vi "Periodic Tasks.vi"(8 "error in":errorcluster) -> ()   [LabVIEW 2016]
doc: "This VI runs in parallel to other tasks. It can contain as many user-defined periodic loops as you need. These can carry out PID or other sorts of timed response."
uses:
  <userlib>/836-libraries/Drive/Drive_Code_V2/Drive_Code_Support/PidClusters/Drive_Code_PID_Bundle.ctl
  <userlib>/836-libraries/Drive/Drive_Code_V2/Drive_Code_Support/Command_Sends/Drive_Code_Command_List.ctl
  <userlib>/836-libraries/Drive/Drive_Code_V2/Drive_Code_Support/SensorTypedefs/Sensor_Cluster.ctl
  <userlib>/836-libraries/Drive/Drive_Code_V2/Drive_Code_Support/SensorTypedefs/Camera_Cluster.ctl
  <vilib>/Rock Robotics/WPI/RobotDrive/WPI_RobotDriveDevRef.ctl
  <vilib>/Rock Robotics/WPI/MotorControl/WPI_MotorControlDeviceRef.ctl
  <vilib>/Rock Robotics/WPI/MotorControl/WPI_MotorControlType.ctl
  <vilib>/Rock Robotics/SystemInterfaces/DIO/FPGA_DIOPWMChannel.ctl
  <vilib>/Rock Robotics/WPI/PWM/WPI_PWMDeadband.ctl
  <userlib>/836-libraries/Drive/Drive_Code_V2/Drive_Code_Support/DriveTrains/Drive_Trains.ctl
  <userlib>/836-libraries/Drive/Drive_Code_V2/Drive_Code_Support/Command_Sends/Drive_Code_Command_Type.ctl
  <userlib>/836-libraries/Drive/Drive_Code_V2/Drive_Code_Support/PidClusters/PidInversions.ctl
  <vilib>/Platform/TimedLoop/XDataNode/timing_clust.ctl
  <vilib>/Platform/TimedLoop/XDataNode/nitl_modes.ctl
  <vilib>/Platform/TimedLoop/XDataNode/wakeup.ctl
  <vilib>/Rock Robotics/WPI/Utilities/WPI_GetSetVariantRefNum.vi
  <userlib>/836-libraries/Drive/Drive_Code_V2/Drive_Code_Support/Command_Sends/Drive_Cmd_Cheesey_Drive.vi
  <userlib>/836-libraries/Drive/Drive_Code_V2/Drive_Code_Support/Command_Sends/Drive_Cmd_Drive_Continuous.vi
  <userlib>/836-libraries/Drive/Drive_Code_V2/Drive_Code_Support/Command_Sends/Drive_Cmd_Turn.vi
  <userlib>/836-libraries/Drive/Drive_Code_V2/Drive_Code_Support/Command_Sends/Drive_Cmd_Drive_Distance.vi
  <userlib>/836-libraries/Drive/Drive_Code_V2/Drive_Code_Support/Command_Sends/Drive_Cmd_Hold_Position.vi
  <userlib>/836-libraries/Drive/Drive_Code_V2/Drive_Code_Support/Command_Sends/Drive_Cmd_Hold_Yaw.vi
  <userlib>/836-libraries/Drive/Drive_Code_V2/Drive_Code_Support/Command_Sends/Drive_Cmd_PID_Update.vi
  <userlib>/836-libraries/Drive/Drive_Code_V2/Drive_Code_Support/Command_Sends/Drive_Cmd_Update_Period.vi
  <userlib>/836-libraries/Drive/Drive_Code_V2/Drive_Code_Support/Command_Sends/Drive_Cmd_Update_PID_Inversion.vi
  <vilib>/platform/TimedLoop/XDataNode/XDataNode.xnode
  <vilib>/Platform/TimedLoop/XDataNode/XDNodeRunTimeDep.lvlib
panel:
  out "SensorFinishedLate":bool
  out "Drive Finished Late":bool
  in  "Tab Control":enum32{"Drive", "Sensors"}(tab)
  out "Distance Error":dbl(knob) scale=0.0..3.0
  out "Turn Error":dbl(knob) scale=0.0..3.0
  in  "Distance Absolute?":bool
  in  "Desired Distance":dbl
  in  "Angle Absolute?":bool
  in  "Desired Angle":dbl
  in  "Max Distance Power":dbl(knob) scale=0.0..1.0
  in  "Max Turn Power":dbl(knob) scale=0.0..1.0
  out "PID Response Turn":cluster{"Yaw":dbl, "Desired Angle":dbl}(graph)
  out "PID Response Distance":cluster{"Distance":dbl, "Desired Distance":dbl}(graph)
  in  "PID Gains":T1={"Yaw, Driving Straight"={"proportional gain (Kc)"=0.025, "integral time (Ti, min)"=0.0, "derivative time (Td, min)"=0.0}, "Yaw, Holding Still"={"proportional gain (Kc)"=0.027, "integral time (Ti, min)"=0.0125, "derivative time (Td, min)"=0.0}, "Distance, Driving Straight"={"proportional gain (Kc)"=1.0, "integral time (Ti, min)"=0.5, "derivative time (Td, min)"=0.0}, "Distance, Holding Still"={"proportional gain (Kc)"=1.0, "integral time (Ti, min)"=0.01, "derivative time (Td, min)"=0.0}}
  in  "Command":T2
  in  "Yaw PID Inverted?":bool
  in  "Distance PID Inverted?":bool
  out "Roll":dbl(graph)
  out "Pitch":dbl(graph)
  out "Yaw":dbl(graph)
  out "Distance":dbl(graph)
  in  "Read Enable":T3={"Cal Status"=TRUE, "Orientation"=TRUE, "Gyro"=FALSE, "Accelerometer"=FALSE, "Quanterion"=FALSE, "Accel Mode"=enum."Linear", "Magnetometer"=FALSE, "Register Mode"=enum."Quaternion"}
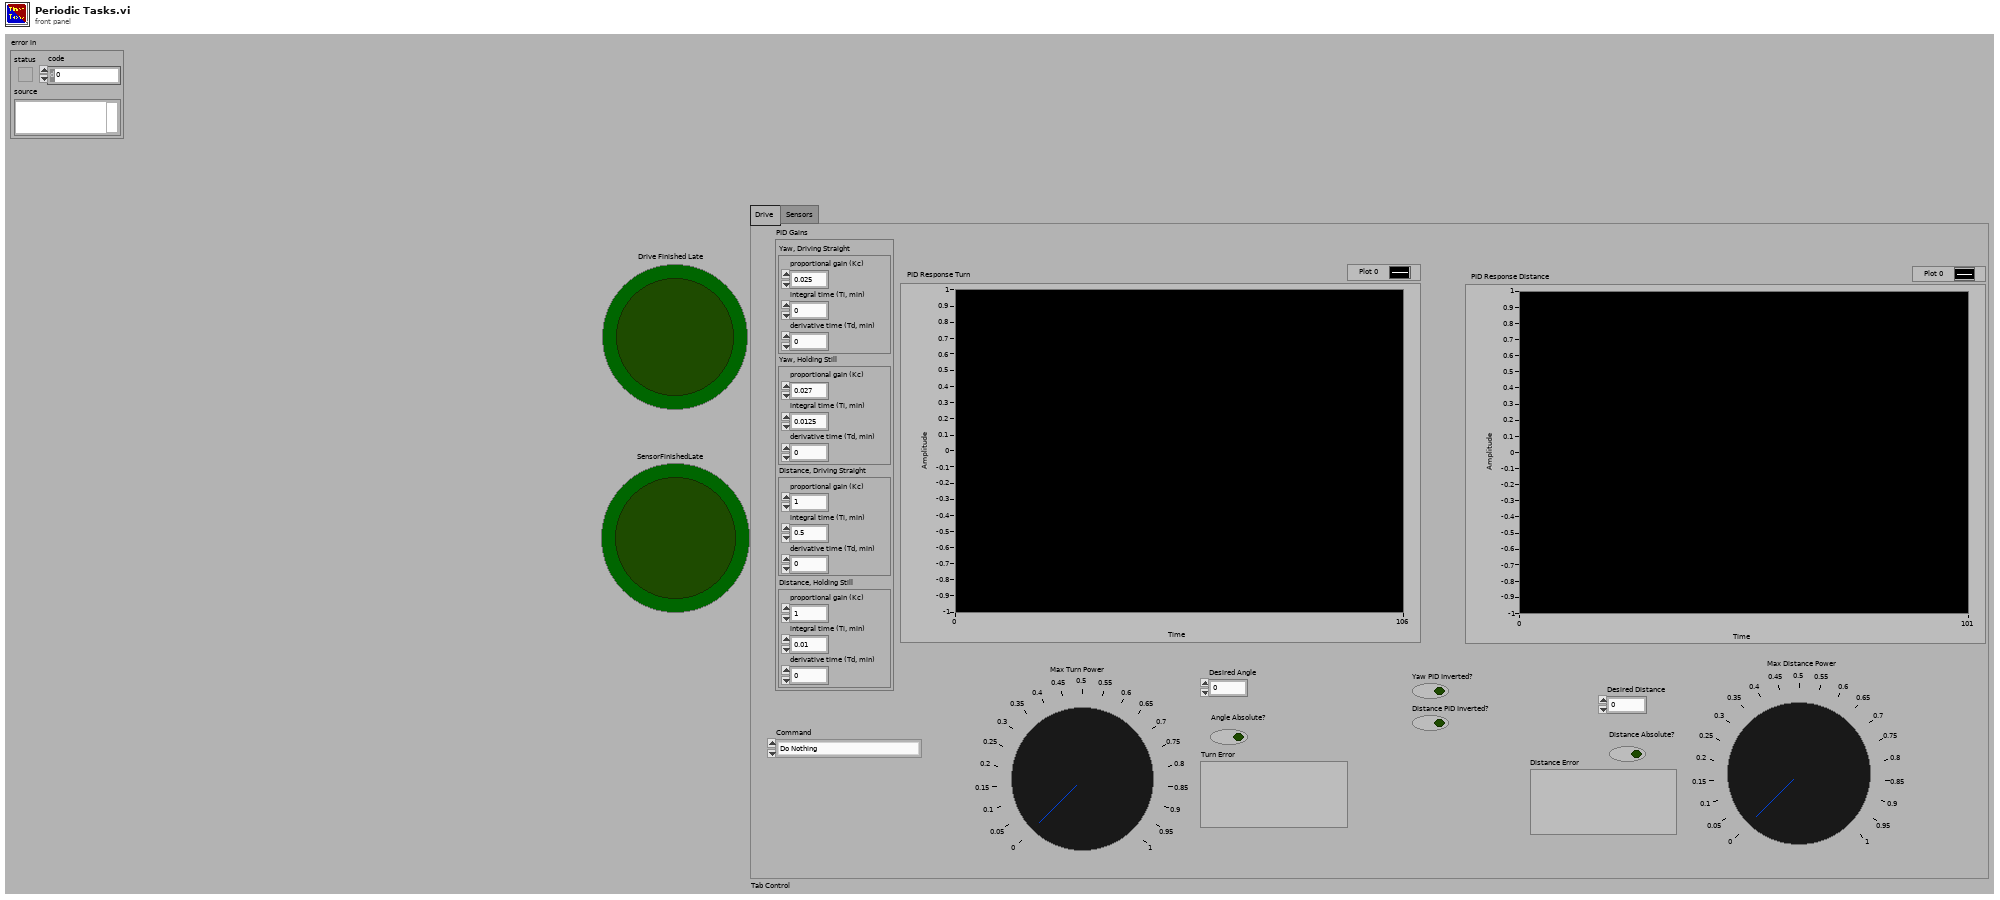
[diagram p1: front panel]
types:
  T1 = typedef "Drive_Code_PID_Bundle.ctl" = cluster{"Yaw, Driving Straight":cluster{"proportional gain (Kc)":dbl, "integral time (Ti, min)":dbl, "derivative time (Td, min)":dbl}, "Yaw, Holding Still":cluster{"proportional gain (Kc)":dbl, "integral time (Ti, min)":dbl, "derivative time (Td, min)":dbl}, "Distance, Driving Straight":cluster{"proportional gain (Kc)":dbl, "integral time (Ti, min)":dbl, "derivative time (Td, min)":dbl}, "Distance, Holding Still":cluster{"proportional gain (Kc)":dbl, "integral time (Ti, min)":dbl, "derivative time (Td, min)":dbl}}
  T2 = typedef "Drive_Code_Command_List.ctl" = enum16{"Do Nothing", "Tank Drive", "Drive Continuous", "Turn", "Drive Distance", "Hold Position", "Hold Yaw", "Follow Camera", "Turn to Camera", "Approach Camera", "PID Update", "Cheesy Drive", "Update Period", "Update PID Inversions"}
  T3 = cluster{"Cal Status":bool, "Orientation":bool, "Gyro":bool, "Accelerometer":bool, "Quanterion":bool, "Accel Mode":enum8{"Raw Data", "Linear", "Gravity"}, "Magnetometer":bool, "Register Mode":enum8{"Euler", "Quaternion"}}
  T4 = typedef "Sensor_Cluster.ctl" = cluster{"Gyro Data":cluster{"Gyro RT FIFO":refnum<k33>, "Gyro Current":dbl, "Gyro Hold":dbl}, "Encoder Data":cluster{"Encoder RT FIFO":refnum<k33>, "Encoder Current":dbl, "Encoder Hold":dbl}, "Camera Data":cluster{"Camera RT FIFO":refnum<k33>, "Camera Current":T5}}
  T5 = typedef "Camera_Cluster.ctl" = cluster{" Angle":dbl, "Valid":bool}
  T6 = typedef "WPI_RobotDriveDevRef.ctl" = cluster{"DevStatus":errorcluster, "Motors[]":T7[], "Square Inputs":bool, "Max Output":dbl}
  T7 = typedef "WPI_MotorControlDeviceRef.ctl" = cluster{"DeviceStatus":errorcluster, "Type":T8, "PWM":cluster{"PWM Channel":T9, "DeadBand":T10}, "CAN":cluster{"Device Number":u8, "SetOutput VI Ref":variant, "GetOutput VI Ref":variant, "Enable VI Ref":variant, "Disable VI Ref":variant, "Data":variant}, "Invert":bool}
  T8 = typedef "WPI_MotorControlType.ctl" = enum16{"PWM", "CAN"}
  T9 = typedef "FPGA_DIOPWMChannel.ctl" = enum8{"PWM 0", "PWM 1", "PWM 2", "PWM 3", "PWM 4", "PWM 5", "PWM 6", "PWM 7", "PWM 8", "PWM 9", "PWM MXP 0", "PWM MXP 1", "PWM MXP 2", "PWM MXP 3", "PWM MXP 4", "PWM MXP 5", "PWM MXP 6", "PWM MXP 7", "PWM MXP 8", "PWM MXP 9", "Invalid"}
  T10 = typedef "WPI_PWMDeadband.ctl" = cluster{"Name":string, "maxPositivePwm":i32, "minPositivePwm":i32, "centerPwm":i32, "maxNegativePwm":i32, "minNegativePwm":i32, "angularRange":u16}
  T11 = typedef "Drive_Trains.ctl" = enum16{"Tank Drive 2 Motor", "Tank Drive 4 Motor", "Mecanum Drive", "Kiwi Drive"}
  T12 = typedef "PidInversions.ctl" = cluster{"Distance PID Inverted?":bool, "Yaw PID Inverted?":bool}
  T13 = cluster{"Sensor Data":T4, "RobotDriveDevRef":T6, "Drive Train":T11, "Valid Commands":bool[], "Drive Comand Notifier":refnum<notifier>, "Command Finished?":refnum<k4>, "Command Canceled":refnum<k4>, "PID Inversions":T12}
  T14 = typedef "WPI_JoystickDevRef.ctl" = cluster{"Device":T15}
  T15 = typedef "WPI_JoystickDeviceEnum.ctl" = enum16{"USB 0", "USB 1", "USB 2", "USB 3", "USB 4", "USB 5"}
  T16 = typedef "XDNodeRunTimeDep.lvlib/timing_clust.ctl" = cluster{"Expected End [f-1]":u64, "Actual End [f-1]":u64, "Finished Late? [f-1]":bool, "Expected End [i-1]":u64, "Actual End [i-1]":u64, "Finished Late? [i-1]":bool, "Expected Start [i]":u64, "Actual Start [i]":u64, "Expected Start [f]":u64, "Actual Start [f]":u64, "Source Name":string, "Structure Name":string, "Period":i64, "Deadline":i64, "Offset":i64, "Start":i64, "Priority":i32, "Timeout":i32, "Mode":T17, "Wakeup Reason":T18, "Error":errorcluster, "Source Type":string, "Secondary Source Type":string, "Global End Time":u64, "Global Start Time":u64, "Frame Duration":u64, "Iteration Duration":u64, "Assigned CPU":i32, "I/O Scan Engine Mode":u32}
  T17 = typedef "XDNodeRunTimeDep.lvlib/nitl_modes.ctl" = enum32{"No Change", "Process missed periods, maintain original phase", "Discard missed periods, maintain original phase", "Process missed periods, ignore original phase", "Discard missed periods, ignore original phase"}
  T18 = typedef "XDNodeRunTimeDep.lvlib/wakeup.ctl" = enum32{"Normal", "Aborted", "Asynchronous wakeup", "Timing source error", "Timed loop error", "Timeout"}
  T19 = typedef "WPI_I2CDevRef.ctl" = cluster{"DevStatus":errorcluster, "Device Address":u8, "Handle":i32, "I2C Bus":T20}
  T20 = typedef "i2c_bus.ctl" = enum16{"I2C On-Board", "I2C MXP", "Invalid"}
  T21 = typedef "WPI_EncoderDevRef.ctl" = cluster{"DevStatus":errorcluster, "EncoderIndex":T22, "CounterIndex":T23, "DistancePerCount":dbl, "Decoding Type":T24}
  T22 = typedef "FPGA_EncoderIdx.ctl" = enum8{"Enc 0", "Enc 1", "Enc 2", "Enc 3", "Enc 4", "Enc 5", "Enc 6", "Enc 7", "Invalid"}
  T23 = typedef "FPGA_CounterCtrSystemIndex.ctl" = enum8{"Ctr 0", "Ctr 1", "Ctr 2", "Ctr 3", "Ctr 4", "Ctr 5", "Ctr 6", "Ctr 7", "Invalid"}
  T24 = typedef "WPI_EncoderType.ctl" = enum16{"1x", "2x", "4x"}
  T25 = cluster{"Yaw":dbl, "Roll":dbl, "Pitch":dbl, "Yaw Wind":dbl, "Roll Wind":dbl, "Pitch Wind":dbl}
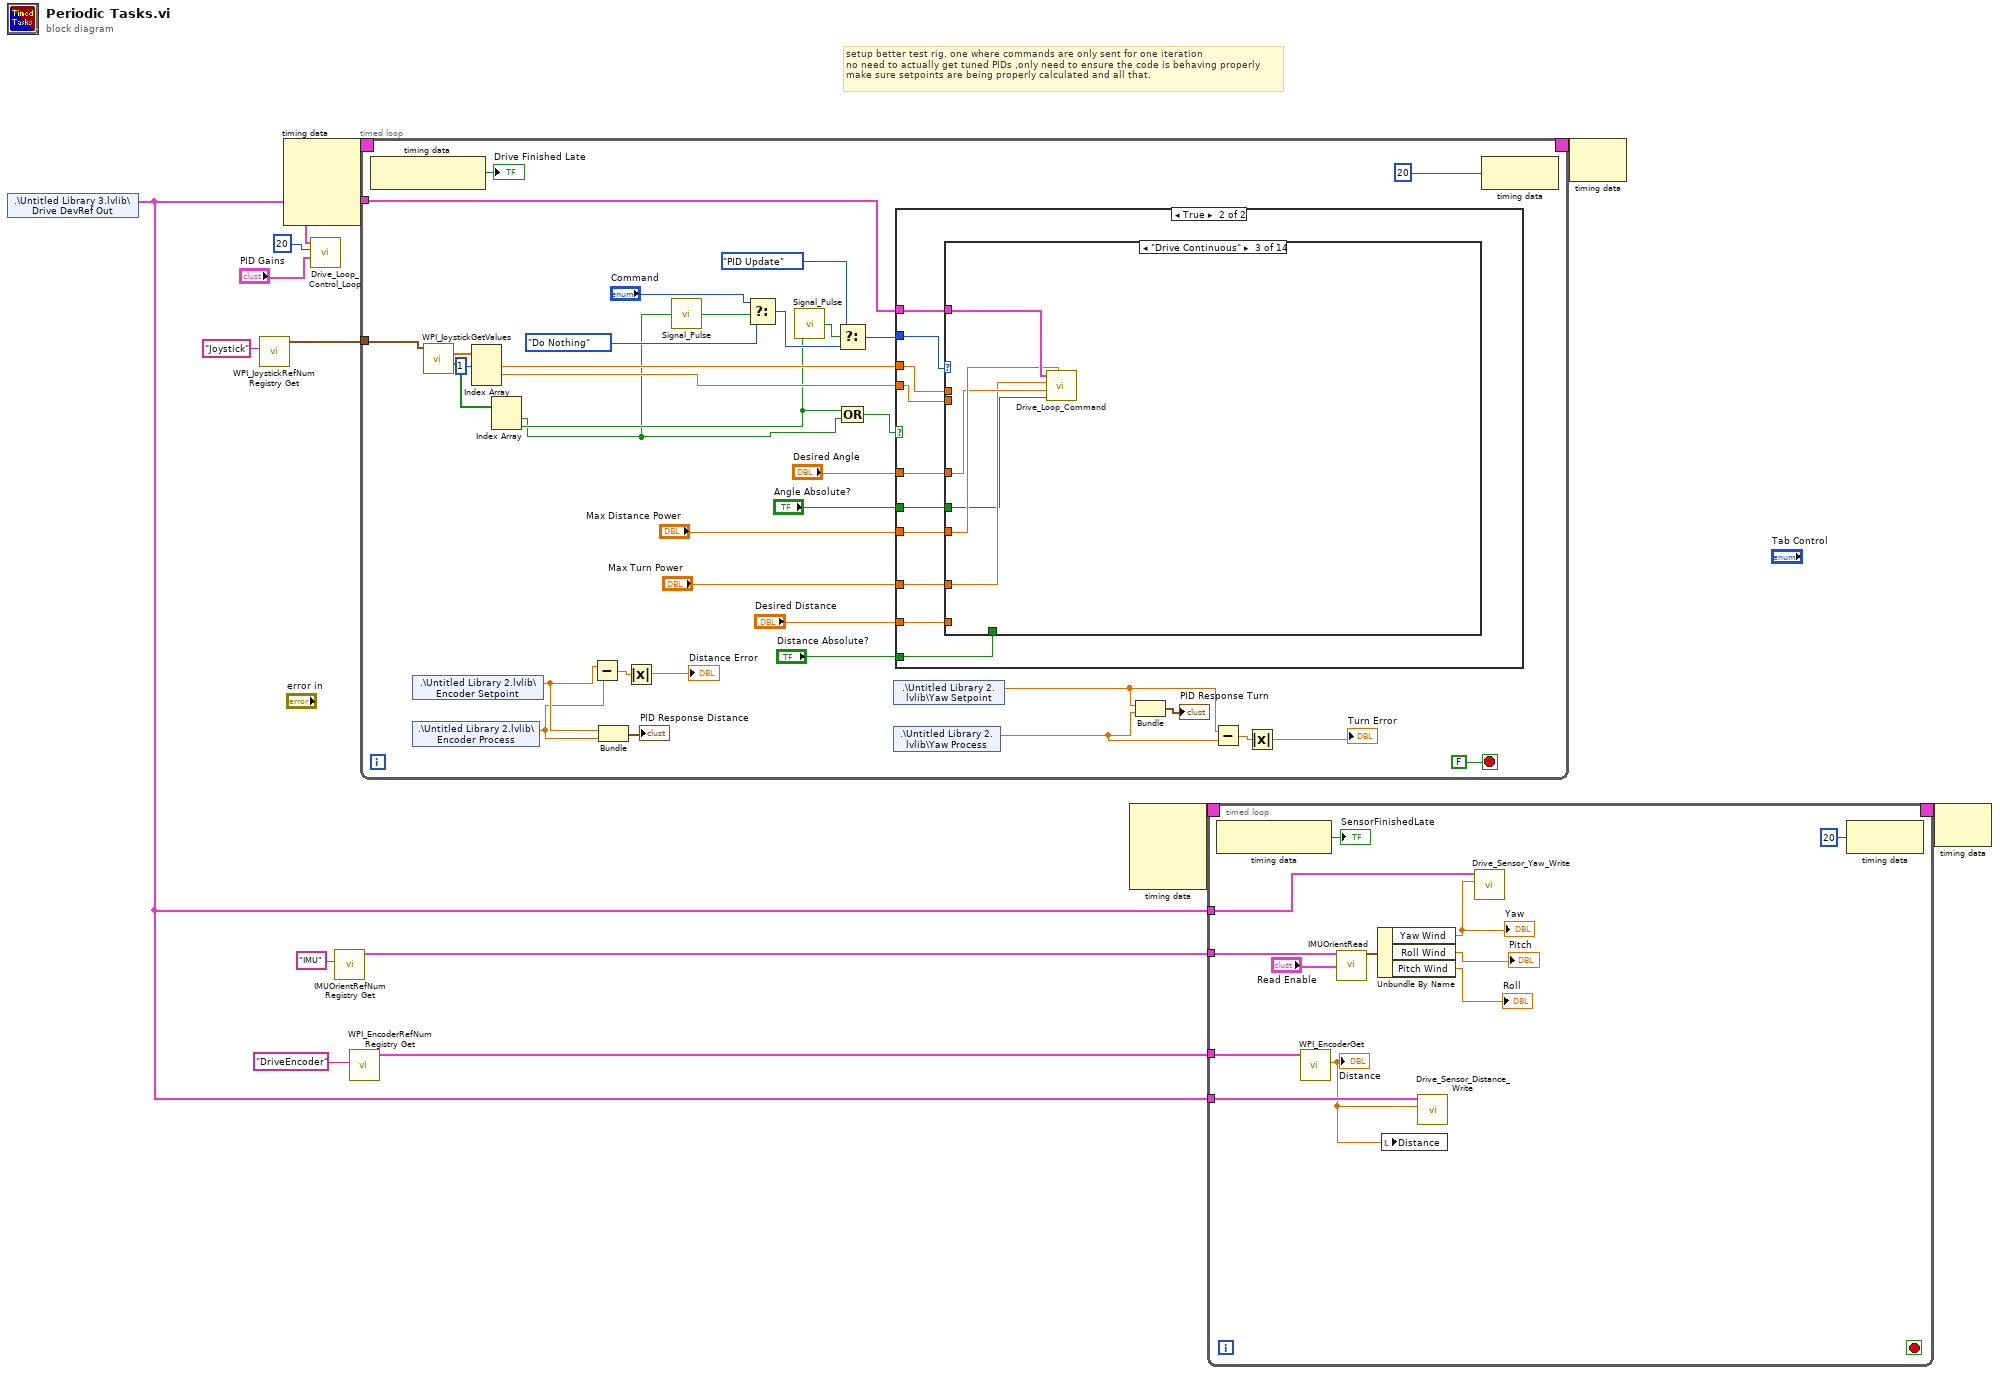
[diagram p0: block diagram]
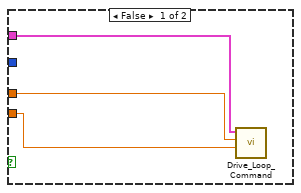
[diagram p2: hidden frame]
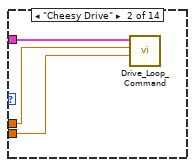
[diagram p4: hidden frame]
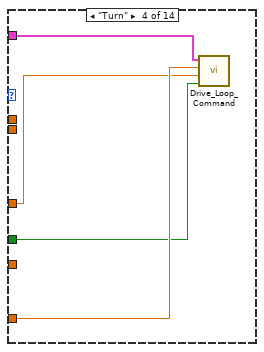
[diagram p5: hidden frame]
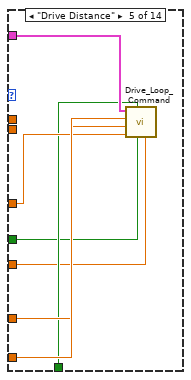
[diagram p6: hidden frame]
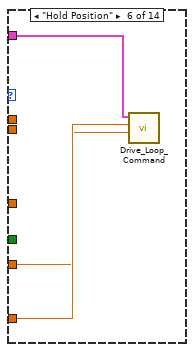
[diagram p7: hidden frame]
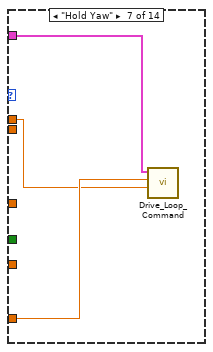
[diagram p8: hidden frame]
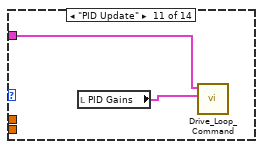
[diagram p12: hidden frame]
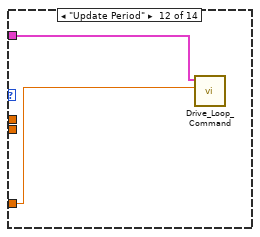
[diagram p13: hidden frame]
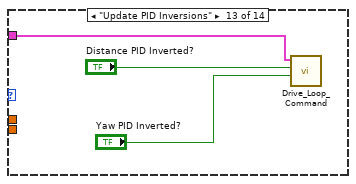
[diagram p14: hidden frame]
diagram:
  # "setup better test rig. one where commands are only sent for one iteration\nno need to actually get tuned PIDs ,only need to ensure the code is behaving properly\nmake sure setpoints are being properly calculated and all that."
  n1 = shared-variable ".\\Untitled Library 3.lvlib\\Drive DevRef Out"() -> (w3:T13)  [unwired: 1 in, 1 out]
  n2 = call <vilib>:"WPI_JoystickRefNum Registry Get.vi"("refnum name"="Joystick") -> ("JoystickDevRef"=w12:T14)  [unwired: 9 in, 1 out]
  n3 = node-c288() -> (w2:T16)  [unwired: 4 in]
  n4 = call <userlib>:"Drive_Loop_Control_Loop.vi"("Init PID Gains"="PID Gains", "Init Period"=i64 20, "Drive DevRef In"=w3) -> ()  [unwired: 9 in]
  n5 = call <userlib>:"IMUOrientRefNum Registry Get.vi"("refnum name"="IMU") -> ("I2CDevRef out"=w6:T19)  [unwired: 9 in, 1 out]
  n6 = call <vilib>:"WPI_EncoderRefNum Registry Get.vi"("refnum name"="DriveEncoder") -> ("EncoderDevRef"=w4:T21)  [unwired: 9 in, 1 out]
  n7 = timed-loop {
    tunnel: w3 -> [w48]
    tunnel: w12 -> [w47]
    timing: w2 -> [_]
    timing-out: [_] -> w1
    stop <- FALSE stop-if-true
    n8 = node-c288() -> (→"Drive Finished Late":bool)  [unwired: 1 in]
    n9 = shared-variable ".\\Untitled Library 2.lvlib\\Encoder Setpoint"() -> (w28:dbl)  [unwired: 1 in, 1 out]
    n10 = shared-variable ".\\Untitled Library 2.lvlib\\Encoder Process"() -> (w27:dbl)  [unwired: 1 in, 1 out]
    n11 = call <vilib>:"WPI_JoystickGetValues.vi"("JoystickDevRef"=w47) -> ("Buttons"=w42:bool[], "Axes"=w46:dbl[])  [unwired: 6 in, 3 out]
    n12 = Index Array(array=w46, index #1=1 ("index")) -> (element #1=w41:dbl, element #2=w40:dbl)  [unwired: 2 in, 1 out]
    n13 = Index Array(array=w42) -> (element #1=w15:bool, element #2=w16:bool)  [unwired: 2 in]
    n14 = Subtract(x=w28, y=w27) -> (x-y=w26:dbl)
    n15 = Bundle("Double"=w28, "Double"=w27) -> (→"PID Response Distance":cluster{"Double":dbl, "Double":dbl})  [unwired: 1 in]
    n16 = Absolute Value(x=w26) -> (abs(x)=→"Distance Error":dbl)
    n17 = call <userlib>:"Signal_Pulse.vi"("Input"=w15) -> ("Output"=w39:bool)
    n18 = Select(t="Command", s=w39, f=Drive_Code_Command_List."Do Nothing") -> (s? t:f=w22:T2)
    n19 = call <userlib>:"Signal_Pulse.vi"("Input"=w16) -> ("Output"=w21:bool)
    n20 = Select(t=Drive_Code_Command_List."PID Update", s=w21, f=w22) -> (s? t:f=w19:T2)
    n21 = Compound Arithmetic op=OR(w16, w15) -> (w14:bool)
    n22 = shared-variable ".\\Untitled Library 2.lvlib\\Yaw Setpoint"() -> (w24:dbl)  [unwired: 1 in, 1 out]
    n23 = shared-variable ".\\Untitled Library 2.lvlib\\Yaw Process"() -> (w23:dbl)  [unwired: 1 in, 1 out]
    n24 = case shown="True" w14 {
      tunnel: w48 -> [w52 w62]
      tunnel: w41 -> [w51 w55]
      tunnel: w40 -> [w50 w54]
      tunnel: "Max Turn Power" -> [_ w61]
      tunnel: "Max Distance Power" -> [_ w60]
      tunnel: "Desired Angle" -> [_ w59]
      tunnel: "Angle Absolute?" -> [_ w58]
      tunnel: "Desired Distance" -> [_ w57]
      tunnel: "Distance Absolute?" -> [_ w56]
      tunnel: w19 -> [_ w53]
      frame False {
        n25 = call-poly <userlib>:"Drive_Loop_Command.vi"("Wheel"=w50, "Throttle"=w51, "Drive Loop Cluster"=w52) -> ()  [unwired: 8 in, 1 out]
      }
      frame True {
        n26 = case shown="\"Drive Continuous\"" w53 {
          tunnel: w62 -> [_ w65 w70 w74 w81 w84 w87 _ _ _ w89 w91 w94 _]
          tunnel: w61 -> [_ _ w67 w73 w79 w83 w86 _ _ _ _ _ _ _]
          tunnel: w60 -> [_ _ w69 _ w75 w82 _ _ _ _ _ _ _ _]
          tunnel: w59 -> [_ _ w68 w72 w78 _ _ _ _ _ _ w90 _ _]
          tunnel: w58 -> [_ _ w66 w71 w76 _ _ _ _ _ _ _ _ _]
          tunnel: w57 -> [_ _ _ _ w80 _ _ _ _ _ _ _ _ _]
          tunnel: w56 -> [_ _ _ _ w77 _ _ _ _ _ _ _ _ _]
          tunnel: w55 -> [_ w64 _ _ _ _ w85 _ _ _ _ _ _ _]
          tunnel: w54 -> [_ w63 _ _ _ _ _ _ _ _ _ _ _ _]
          frame "Do Nothing", Default {
          }
          frame "Cheesy Drive" {
            n27 = call-poly <userlib>:"Drive_Loop_Command.vi"("Wheel"=w63, "Throttle"=w64, "Drive Loop Cluster"=w65) -> ()  [unwired: 8 in, 1 out]
          }
          frame "Drive Continuous" {
            n28 = call-poly <userlib>:"Drive_Loop_Command.vi"("Foward Power"=w69, "Absolute Angle?"=w66, "Angle"=w68, "Max Turn Power"=w67, "Drive Loop Cluster"=w70) -> ()  [unwired: 6 in, 1 out]
          }
          frame "Turn" {
            n29 = call-poly <userlib>:"Drive_Loop_Command.vi"("Angle Abolute?"=w71, "Angle"=w72, "Max Power"=w73, "Drive Loop Cluster"=w74) -> ()  [unwired: 7 in, 1 out]
          }
          frame "Drive Distance" {
            n30 = call-poly <userlib>:"Drive_Loop_Command.vi"("Max Forward Power"=w75, "Absolute Angle?"=w76, "Absolute Distance?"=w77, "Angle"=w78, "Max Turn Power"=w79, "Distance"=w80, "Drive Loop Cluster"=w81) -> ()  [unwired: 4 in, 1 out]
          }
          frame "Hold Position" {
            n31 = call-poly <userlib>:"Drive_Loop_Command.vi"("Max Forward Power"=w82, "Max Turn Power"=w83, "Drive Loop Cluster"=w84) -> ()  [unwired: 8 in, 1 out]
          }
          frame "Hold Yaw" {
            n32 = call-poly <userlib>:"Drive_Loop_Command.vi"("Forward Power"=w85, "Max Turn Power"=w86, "Drive Loop Cluster"=w87) -> ()  [unwired: 8 in, 1 out]
          }
          frame "Follow Camera" {
          }
          frame "Turn to Camera" {
          }
          frame "Approach Camera" {
          }
          frame "PID Update" {
            n33 = local read "PID Gains"() -> (w88:T1)
            n34 = call-poly <userlib>:"Drive_Loop_Command.vi"("PID Gains"=w88, "Control Cluster"=w89) -> ()  [unwired: 10 in]
          }
          frame "Update Period" {
            n35 = call-poly <userlib>:"Drive_Loop_Command.vi"("Period"=w90, "DriveDevRefIn"=w91) -> ()  [unwired: 10 in]
          }
          frame "Update PID Inversions" {
            n36 = call-poly <userlib>:"Drive_Loop_Command.vi"("Yaw PID Inverted?"="Yaw PID Inverted?", "Distance PID Inverted?"="Distance PID Inverted?", "DriveDevRefIn"=w94) -> ()  [unwired: 9 in]
          }
          frame "Tank Drive" {
          }
        }
      }
    }
    n37 = Bundle("Double"=w24, "Double"=w23) -> (→"PID Response Turn":cluster{"Double":dbl, "Double":dbl})  [unwired: 1 in]
    n38 = Subtract(x=w24, y=w23) -> (x-y=w25:dbl)
    n39 = Absolute Value(x=w25) -> (abs(x)=→"Turn Error":dbl)
    n40 = node-c288(i64 20 ("Period")) -> ()  [unwired: 1 out]
  }
  n41 = node-c288() -> (w11:T16)  [unwired: 4 in]
  n42 = timed-loop {
    timing: w11 -> [_]
    timing-out: [_] -> w10
    tunnel: w6 -> [w110]
    tunnel: w4 -> [w105]
    tunnel: w3 -> [w104]
    tunnel: w3 -> [w103]
    stop <- _ stop-if-true
    n43 = node-c288() -> (→"SensorFinishedLate":bool)  [unwired: 1 in]
    n44 = call <vilib>:"WPI_EncoderGet.vi"("EncoderDevRef"=w105) -> ("Distance"=w101:dbl)  [unwired: 5 in, 5 out]
    "Distance" <- w101
    n45 = call <userlib>:"IMUOrientRead.vi"("I2CDevRef"=w110, "Read Enable"="Read Enable") -> ("Orient Y/R/P"=w108:T25)  [unwired: 7 in, 6 out]
    n46 = Unbundle By Name(w108) -> ("Yaw Wind"=w102:dbl, "Roll Wind"=→"Pitch":dbl, "Pitch Wind"=→"Roll":dbl)
    "Yaw" <- w102
    n47 = local write "Distance"(w101) -> ()
    n48 = call <userlib>:"Drive_Sensor_Distance_Write.vi"("Distance"=w101, "Drive DevRef In"=w104) -> ()  [unwired: 10 in]
    n49 = call <userlib>:"Drive_Sensor_Yaw_Write.vi"("Angle"=w102, "Drive DevRef In"=w103) -> ()  [unwired: 10 in]
    n50 = node-c288(i64 20 ("Period")) -> ()  [unwired: 1 out]
  }
  n51 = node-c288(w1) -> ()  [unwired: 1 out]
  n52 = node-c288(w10) -> ()  [unwired: 1 out]
